vi "Logfile Paths.vi"() -> (2 "TDMS Logfile path":path, 3 "CSV Logfile path":path)   [LabVIEW 2018, in "TDMS Log.lvlib"]
uses:
  TDMS Log.lvlib
  <vilib>/Utility/sysdir.llb/System Directory Type.ctl
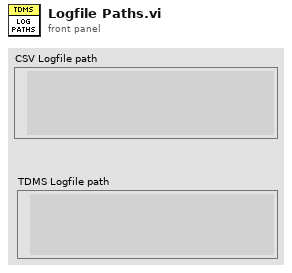
[diagram p1: front panel]
types:
  T1 = typedef "System Directory Type.ctl" = i32
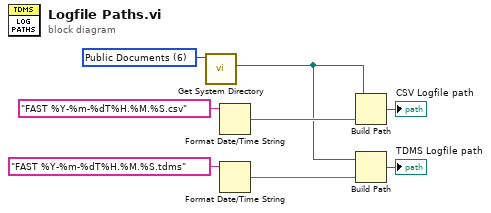
[diagram p0: block diagram]
diagram:
  w7 = T1 6 items=["User Home"=0, "User Desktop"=1, "User Documents"=2, "User Application Data"=3, "User Preferences"=4, "User Temporary"=5, "Public Documents"=6, "Public Application Data"=7, "Public Preferences"=8, "Public Cache"=13, "System Core Libraries"=9, "System Installed Libraries"=10, "Application Files"=11, "Boot Volume Root"=12] ("system directory type")
  n1 = call <vilib>:"Get System Directory.vi"("system directory type"=w7) -> ("system directory"=w1:path)  [unwired: 10 in]
  n2 = Format Date/Time String(time format string (%c)="FAST %Y-%m-%dT%H.%M.%S.csv") -> (date/time string=w6:string)  [unwired: 2 in]
  n3 = Format Date/Time String(time format string (%c)="FAST %Y-%m-%dT%H.%M.%S.tdms") -> (date/time string=w3:string)  [unwired: 2 in]
  n4 = Build Path(base path=w1, name or relative path=w6) -> (appended path=→"CSV Logfile path":path)
  n5 = Build Path(base path=w1, name or relative path=w3) -> (appended path=→"TDMS Logfile path":path)
